vi "数字输入_软件按需单点(端口).vi"() -> ()   [LabVIEW 2013]
doc: "This example demonstrates how to read values from a digital input port."
uses:
  <userlib>/ArtDAQ/_SubVI/ArtDAQ_CreateDIChan.vi
  <userlib>/ArtDAQ/_SubVI/ArtDAQ_Read Digital Bool 1Chan 1Samp(Port).vi
panel:
  out "数据":bool[](array[boolean])
  out "错误输出":errorcluster
  in  "?":bool
  in  "超时(ms)":u32=10
  in  "端口":string="Dev1/port0"
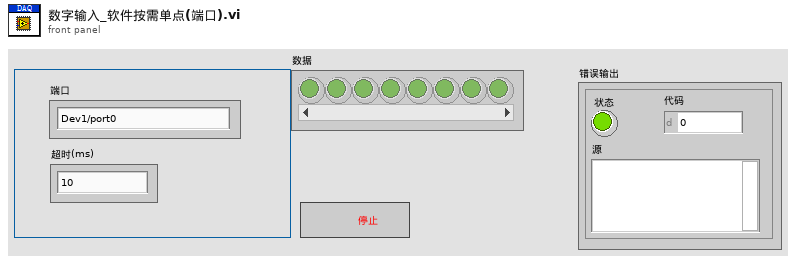
[diagram p1: front panel]
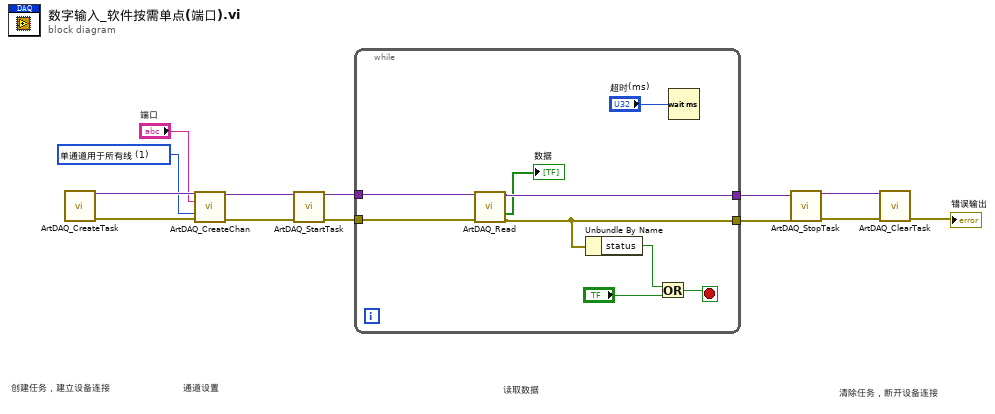
[diagram p0: block diagram]
diagram:
  w3 = 1 items=["单通道用于单条线", "单通道用于所有线"] ("线分组")
  # "清除任务，断开设备连接"
  # "读取数据"
  # "通道设置"
  # "创建任务，建立设备连接"
  n1 = call <userlib>:"ArtDAQ_CreateTask.vi"() -> ("任务句柄"=w13:variant, "错误输出"=w12:errorcluster)  [unwired: 14 in]
  n2 = call-poly <userlib>:"ArtDAQ_CreateChan.vi"("任务句柄"=w13, "线"="端口", "线分组"=w3, "错误输入"=w12) -> ("任务句柄"=w11:variant, "错误输出"=w10:errorcluster)  [unwired: 10 in]
  n3 = call <userlib>:"ArtDAQ_StartTask.vi"("任务句柄"=w11, "错误输入"=w10) -> ("任务句柄"=w9:variant, "错误输出"=w8:errorcluster)  [unwired: 12 in]
  n4 = while {
    tunnel: w9 -> [w18]
    tunnel: w8 -> [w16]
    tunnel: [w17] -> w7
    tunnel: [w15] -> w6
    stop <- w21 stop-if-true
    n5 = call-poly <userlib>:"ArtDAQ_Read.vi"("任务句柄"=w18, "错误输入"=w16) -> ("任务句柄"=w17:variant, "数据"=→"数据":bool[], "错误输出"=w15:errorcluster)  [unwired: 11 in]
    n6 = Unbundle By Name(w15) -> ("status"=w22:bool)
    n7 = Or(x=w22, y="?") -> (x .or. y?=w21:bool)
    n8 = Wait (ms)(milliseconds to wait="超时(ms)") -> ()  [unwired: 1 out]
  }
  n9 = call <userlib>:"ArtDAQ_StopTask.vi"("任务句柄"=w7, "错误输入"=w6) -> ("任务句柄"=w4:variant, "错误输出"=w5:errorcluster)  [unwired: 12 in]
  n10 = call <userlib>:"ArtDAQ_ClearTask.vi"("任务句柄"=w4, "错误输入"=w5) -> ("错误输出"=→"错误输出":errorcluster)  [unwired: 13 in]
